vi "uActor_Exec.vi"(6 "Original uMsg":refnum<class "uMsg.lvclass">, 8 "error in (no error)":errorcluster, 9 "Data":refnum<class "uData.lvclass">, 10 "Command":string, 11 "uObserver in":refnum<class "uObserver.lvclass">) -> (0 "error out":errorcluster, 1 "reply":refnum<class "uData.lvclass">, 3 "uObserver out":refnum<class "uObserver.lvclass">)   [LabVIEW 2023, in "uLib.lvlib" / "uObserver.lvclass"]
doc: "uObserver actor by default ignores any output wired to the output terminal 'reply' in the child override EXEC method unless the child class invokes the uActor_EnableAutoAck method."
uses:
  uObserver.lvclass
  uData/uData/uData.lvclass
  uMsg/uMsg/uMsg.lvclass
  uObserver.lvclass/uObserver.ctl
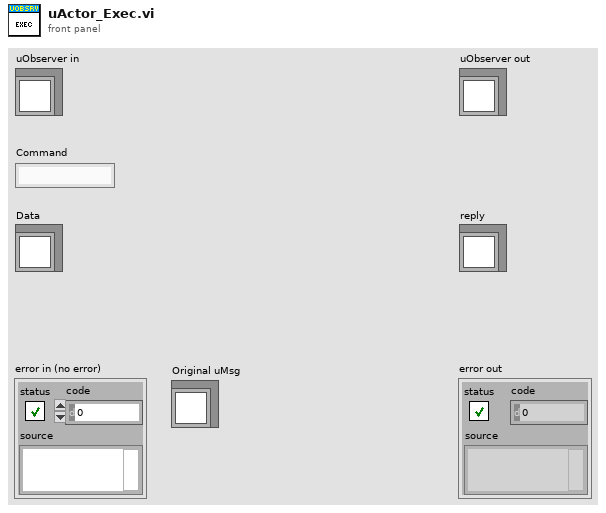
[diagram p1: front panel]
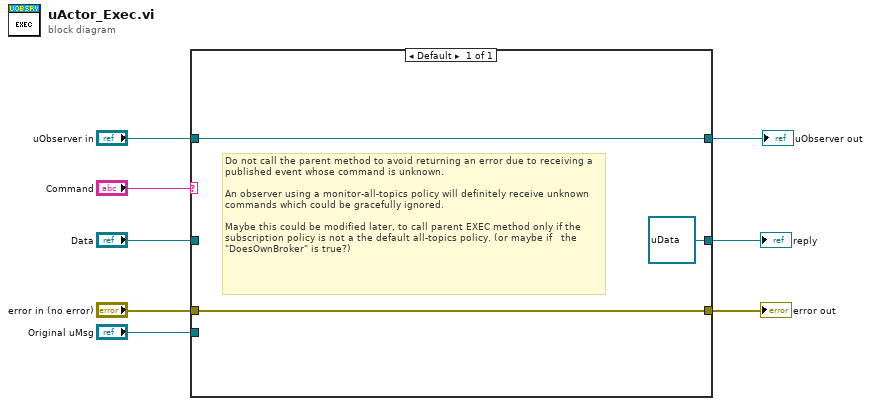
[diagram p0: block diagram]
diagram:
  n1 = case shown="Default" "Command" {
    tunnel: [w11] -> w8
    tunnel: [refnum<class "uData.lvclass"> refnum ("reply")] -> w7
    tunnel: [w10] -> w6
    tunnel: "Original uMsg" -> [_]
    tunnel: "error in (no error)" -> [w11]
    tunnel: "Data" -> [_]
    tunnel: "uObserver in" -> [w10]
    frame Default {
      # "Do not call the parent method to avoid returning an error due to receiving a published event whose command is unknown. \n\nAn observer using a monitor-all-topics policy will definitely receive unknown commands which could be gracefully ignored.\n\nMaybe this could be modified later, to call parent EXEC method only if the subscription policy is not a the default all-topics policy. (or maybe if   the \"DoesOwnBroker\" is true?)"
    }
  }
  "error out" <- w8
  "uObserver out" <- w6
  "reply" <- w7
